vi "AI Continuous FPGA（Host）.vi"() -> ()   [LabVIEW 2019]
uses:
  <vilib>/rvi/interface/nirviOpenFPGA/nirviOpenFPGA.xnode
  <vilib>/rvi/interface/nirviMethod/nirviMethod.xnode
  <vilib>/FPGAPlugInAG/Dynamic/niLvFpga_ConfigureFifo_Dynamic.vi
  <vilib>/rvi/errors/niLvFpgaMergeErrorWithErrorCode.vi
  <vilib>/rvi/interface/nirviReadWriteControl/nirviReadWriteControl.xnode
  <vilib>/FPGAPlugInAG/Dynamic/niLvFpga_ReadFifo_Dynamic.vi
  <vilib>/rvi/interface/nirviCloseFPGA/nirviCloseFPGA.xnode
  <vilib>/FPGAPlugInAG/Dynamic/niLvFpga_Run_Dynamic.vi
  FPGA Bitfiles/aiofpga_FPGATarget_AIContinuousFPGA_w4BGLPLJcoU.lvbitx
  AI Continuous FPGA.vi
  <vilib>/FPGAPlugInAG/ELVIS III/niLvFpga_Open_ELVIS III.vi
  <vilib>/rvi/interface/common/dynamic/niFpgaDynamicAddResources.vi
  NiFpgaLv.dll
  <vilib>/Utility/error.llb/Error Cluster From Error Code.vi
  <vilib>/rvi/interface/Simulation/niFpgaSimulationCallBeginRW.vi
  <vilib>/rvi/errors/niLvFpgaAdjustHostInterfaceError.vi
  <vilib>/FPGAPlugInAG/Dynamic/niLvFpga_Close_Dynamic.vi
  <vilib>/LabVIEW Targets/FPGA/RIO/BlueMoonOnboardIO/nicrio_cRIO-BlueMoonOnboardAi_VoltageRange.ctl
  <vilib>/LabVIEW Targets/FPGA/RIO/BlueMoonOnboardIO/nicrio_cRIO-BlueMoonOnboardAi_TerminalMod.ctl
panel:
  in  "停止":bool
  out "波形图表":dbl[](graph)
  in  "A?B":bool=TRUE
  in  "Sample Number":u32=1000 format="%.0p"
  in  "Channel Number [i + 1]":u8
  in  "Terminal Mode [i + 1]":T1=1 items=["DIFF", "RSE"]
  in  "Voltage Range [i + 1]":T2 items=["+/- 10V", "+/- 5V", "+/- 2V", "+/- 1V"]
  in  "Sample Rate":u32=1000 format="%.0p"
  in  "Start":bool
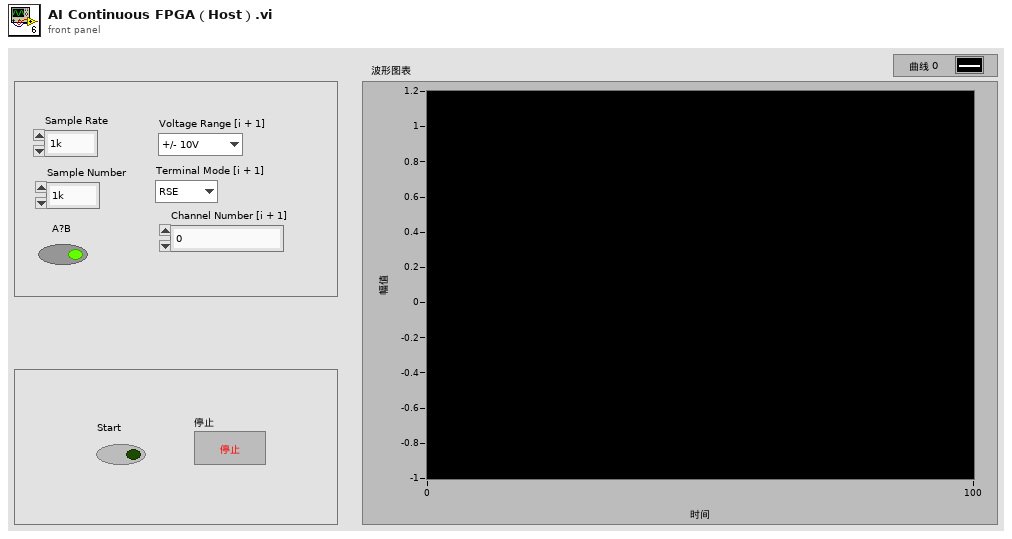
[diagram p1: front panel]
types:
  T1 = typedef "nicrio_cRIO-BlueMoonOnboardAi_TerminalMod.ctl" = u8
  T2 = typedef "nicrio_cRIO-BlueMoonOnboardAi_VoltageRange.ctl" = u8
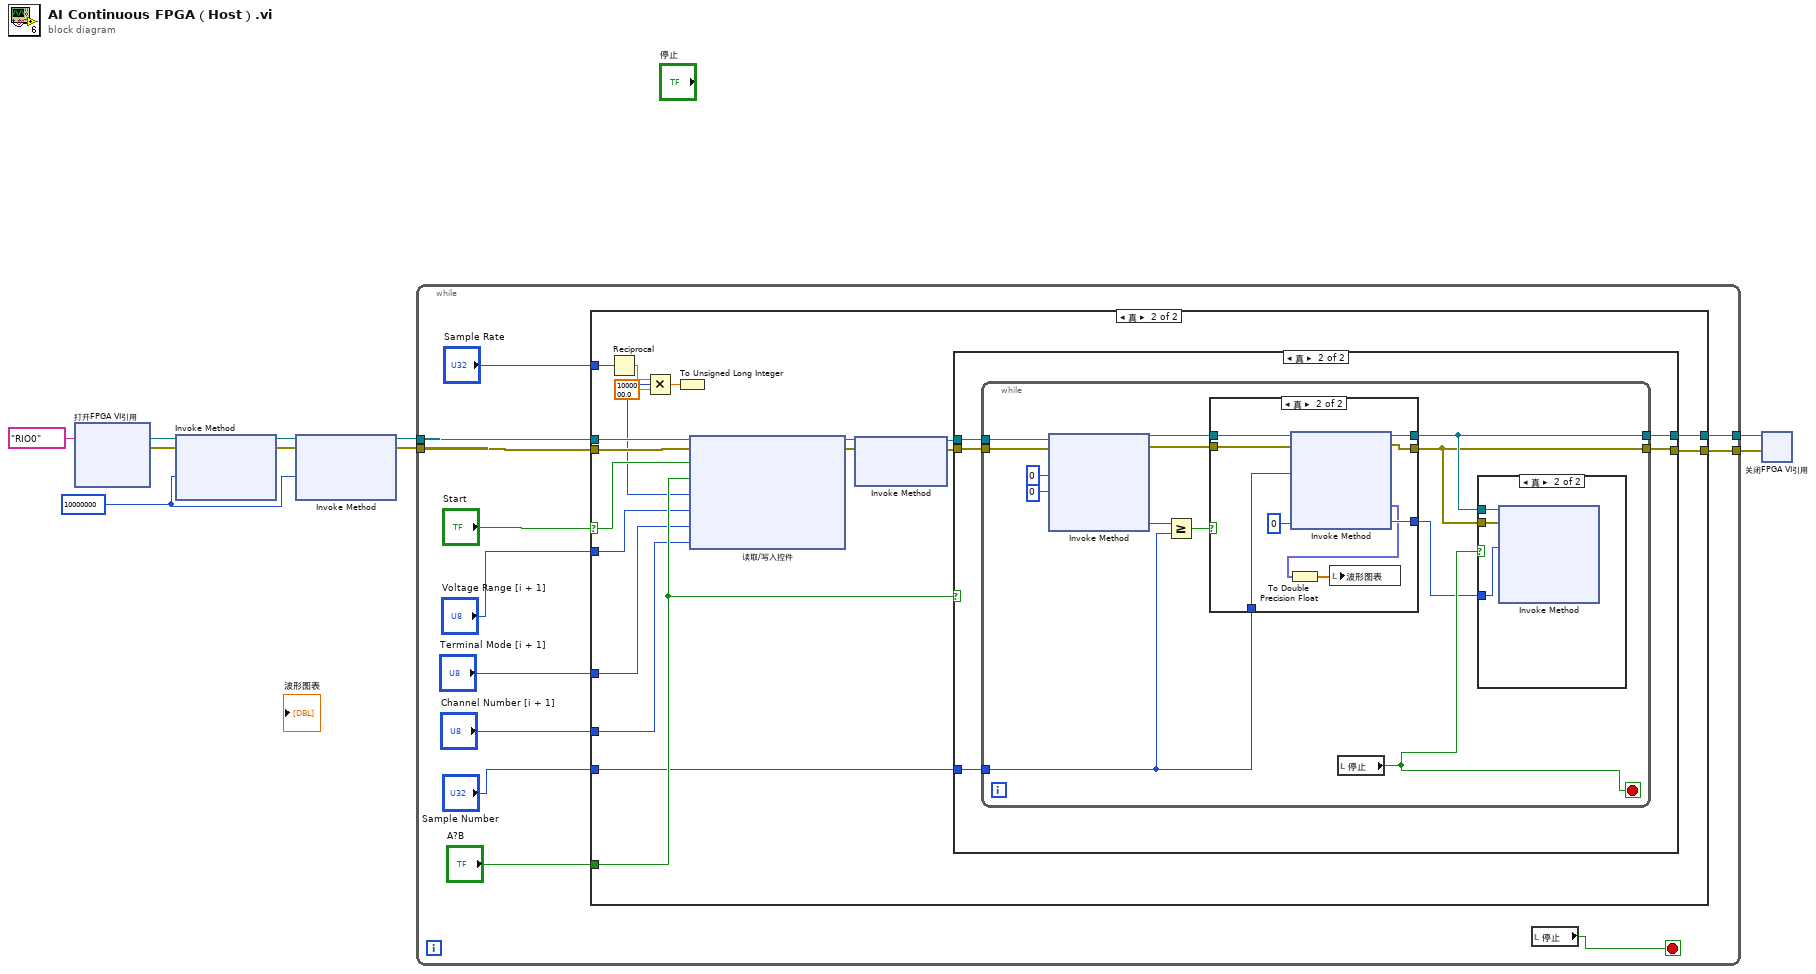
[diagram p0: block diagram]
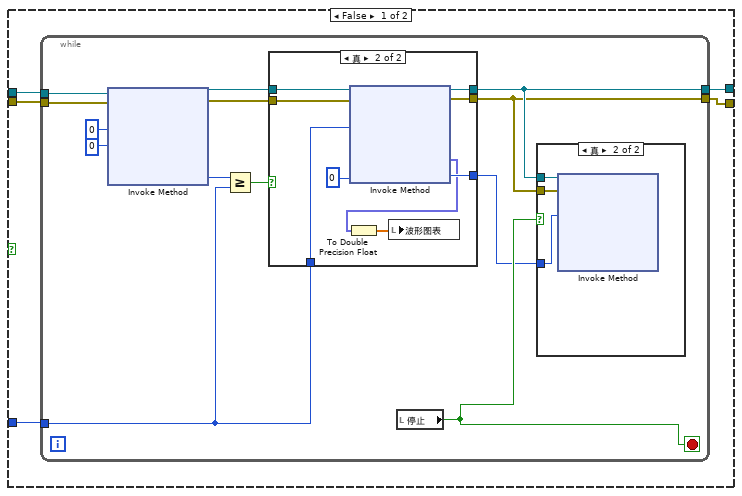
[diagram p3: hidden frame]
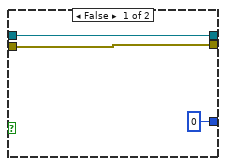
[diagram p5: hidden frame]
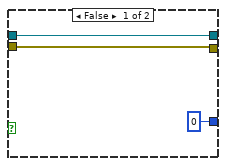
[diagram p7: hidden frame]
diagram:
  w5 = u32 10000000 ("请求的深度")
  n1 = xnode "打开FPGA VI引用"("资源名称"=tag "RIO0") -> ("FPGA VI引用输出"=w9:refnum<k20>, "错误输出"=w8:errorcluster)  [unwired: 1 in]
  n2 = xnode "Invoke Method"("FPGA VI引用输入"=w9, "错误输入"=w8, "请求的深度"=w5) -> ("FPGA VI引用输出"=w6:refnum<k20>, "错误输出"=w7:errorcluster)  [unwired: 1 out]
  n3 = xnode "Invoke Method"("FPGA VI引用输入"=w6, "错误输入"=w7, "请求的深度"=w5) -> ("FPGA VI引用输出"=w1:refnum<k20>, "错误输出"=w2:errorcluster)  [unwired: 1 out]
  n4 = while {
    tunnel: w2 -> [w21]
    tunnel: w1 -> [w20]
    tunnel: [w12] -> w4
    tunnel: [w11] -> w3
    stop <- w13 stop-if-true
    n5 = case shown="真" "Start" {
      selector: "Start" -> [_ w41]
      tunnel: w21 -> [w24 w43]
      tunnel: w20 -> [w23 w42]
      tunnel: "A?B" -> [_ w40]
      tunnel: "Voltage Range [i + 1]" -> [_ w39]
      tunnel: "Terminal Mode [i + 1]" -> [_ w38]
      tunnel: "Channel Number [i + 1]" -> [_ w37]
      tunnel: "Sample Rate" -> [_ w33]
      tunnel: "Sample Number" -> [_ w31]
      tunnel: [w24 w30] -> w12
      tunnel: [w23 w29] -> w11
      frame False {
      }
      frame True {
        n6 = Reciprocal(x=w33) -> (1/x=w36:dbl)
        n7 = Multiply(x=w36, y=1000000.0) -> (x*y=w34:dbl)
        n8 = To Unsigned Long Integer(number=w34) -> (unsigned 32bit integer=w32:u32)
        n9 = xnode "读取/写入控件"("FPGA VI引用输入"=w42, "错误输入"=w43, "Start"=w41, "A?B"=w40, "Sample time"=w32, "Voltage Range [i + 1]"=w39, "Terminal Mode [i + 1]"=w38, "Channel Number [i + 1]"=w37) -> ("FPGA VI引用输出"=w27:refnum<k20>, "错误输出"=w28:errorcluster)
        n10 = xnode "Invoke Method"("FPGA VI引用输入"=w27, "错误输入"=w28) -> ("FPGA VI引用输出"=w25:refnum<k20>, "错误输出"=w26:errorcluster)  [unwired: 1 in]
        n11 = case shown="真" w40 {
          tunnel: w26 -> [w47 w81]
          tunnel: w25 -> [w48 w80]
          tunnel: w31 -> [w46 w79]
          tunnel: [w45 w78] -> w30
          tunnel: [w44 w77] -> w29
          frame False {
            n12 = while {
              tunnel: w47 -> [w60]
              tunnel: w48 -> [w61]
              tunnel: w46 -> [w56]
              tunnel: [w50] -> w44
              tunnel: [w49] -> w45
              stop <- w54 stop-if-true
              n13 = xnode "Invoke Method"("FPGA VI引用输入"=w61, "错误输入"=w60, "元素数量"=u32 0, "超时(ms)"=0) -> ("FPGA VI引用输出"=w52:refnum<k20>, "错误输出"=w53:errorcluster, "剩余元素"=w57:u32)  [unwired: 1 out]
              n14 = Greater Or Equal?(x=w57, y=w56) -> (x >= y?=w55:bool)
              n15 = case shown="真" w55 {
                tunnel: w56 -> [_ w76]
                tunnel: w53 -> [w67 w74]
                tunnel: w52 -> [w66 w73]
                tunnel: [u32 0 ("剩余元素") w72] -> w51
                tunnel: [w67 w71] -> w49
                tunnel: [w66 w70] -> w50
                frame False {
                }
                frame True {
                  n16 = xnode "Invoke Method"("FPGA VI引用输入"=w73, "错误输入"=w74, "元素数量"=w76, "超时(ms)"=0) -> ("FPGA VI引用输出"=w70:refnum<k20>, "错误输出"=w71:errorcluster, "数据"=w68:fxp<+/-,24,5>[], "剩余元素"=w72:u32)
                  n17 = To Double Precision Float(number=w68) -> (double precision float=w69:dbl[])
                  n18 = local write "波形图表"(w69) -> ()
                }
              }
              n19 = local read "停止"() -> (w54:bool)
              n20 = case shown="真" w54 {
                tunnel: w51 -> [_ w62]
                tunnel: w49 -> [_ w64]
                tunnel: w50 -> [_ w63]
                frame False {
                }
                frame True {
                  n21 = xnode "Invoke Method"("FPGA VI引用输入"=w63, "错误输入"=w64, "元素数量"=w62) -> ()  [unwired: 1 in, 4 out]
                }
              }
            }
          }
          frame True {
            n22 = while {
              tunnel: w81 -> [w93]
              tunnel: w80 -> [w94]
              tunnel: w79 -> [w89]
              tunnel: [w83] -> w77
              tunnel: [w82] -> w78
              stop <- w87 stop-if-true
              n23 = xnode "Invoke Method"("FPGA VI引用输入"=w94, "错误输入"=w93, "元素数量"=u32 0, "超时(ms)"=0) -> ("FPGA VI引用输出"=w85:refnum<k20>, "错误输出"=w86:errorcluster, "剩余元素"=w90:u32)  [unwired: 1 out]
              n24 = Greater Or Equal?(x=w90, y=w89) -> (x >= y?=w88:bool)
              n25 = case shown="真" w88 {
                tunnel: w89 -> [_ w109]
                tunnel: w86 -> [w100 w107]
                tunnel: w85 -> [w99 w106]
                tunnel: [u32 0 ("剩余元素") w105] -> w84
                tunnel: [w100 w104] -> w82
                tunnel: [w99 w103] -> w83
                frame False {
                }
                frame True {
                  n26 = xnode "Invoke Method"("FPGA VI引用输入"=w106, "错误输入"=w107, "元素数量"=w109, "超时(ms)"=0) -> ("FPGA VI引用输出"=w103:refnum<k20>, "错误输出"=w104:errorcluster, "数据"=w101:fxp<+/-,24,5>[], "剩余元素"=w105:u32)
                  n27 = To Double Precision Float(number=w101) -> (double precision float=w102:dbl[])
                  n28 = local write "波形图表"(w102) -> ()
                }
              }
              n29 = local read "停止"() -> (w87:bool)
              n30 = case shown="真" w87 {
                tunnel: w84 -> [_ w95]
                tunnel: w82 -> [_ w97]
                tunnel: w83 -> [_ w96]
                frame False {
                }
                frame True {
                  n31 = xnode "Invoke Method"("FPGA VI引用输入"=w96, "错误输入"=w97, "元素数量"=w95) -> ()  [unwired: 1 in, 4 out]
                }
              }
            }
          }
        }
      }
    }
    n32 = local read "停止"() -> (w13:bool)
  }
  n33 = xnode "关闭FPGA VI引用"("FPGA VI引用输入"=w3, "错误输入"=w4) -> ()  [unwired: 1 out]
